vi "Destroy.vi"(8 "error in (no error)":errorcluster, 11 "Numeric In":refnum<class "Numeric.lvclass">) -> (0 "error out":errorcluster, 3 "Numeric Out":refnum<class "Numeric.lvclass">)   [LabVIEW 2017, in "Front Panel Publisher.lvlib" / "Numeric.lvclass"]
uses:
  Numeric.lvclass
  Control_class/Control.lvclass
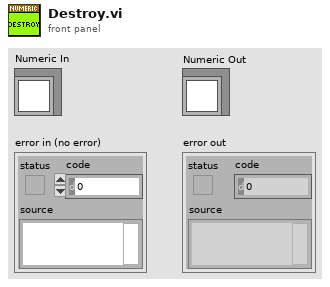
[diagram p1: front panel]
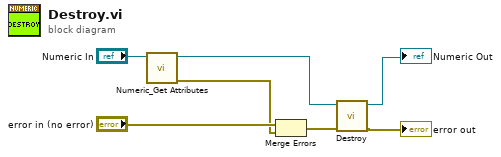
[diagram p0: block diagram]
diagram:
  n1 = call "Numeric_Get Attributes.vi"("Numeric In"="Numeric In") -> ("error out"=w1:errorcluster, "Numeric Out"=w2:refnum<class "Numeric.lvclass">)  [unwired: 8 in, 1 out]
  n2 = Merge Errors("error in (no error)", w1) -> (w5:errorcluster)
  n3 = call-parent "Destroy.vi"("error in (no error)"=w5, "Control In"=w2) -> ("error out"=→"error out":errorcluster, "Control Out"=→"Numeric Out":refnum<class "Numeric.lvclass">)  [unwired: 8 in]
